vi "Next Background Music.vi"(8 "error in (no error)":errorcluster, 9 "Music Paused":bool, 10 "Dyn Sounds Path":path, 11 "Sounds":T1[](array[typedef]) {"Task ID" format="%.0x"}) -> (0 "error out":errorcluster, 3 "Sounds Out":T1[](array[typedef]) {"Task ID" format="%.0x"}, 5 "BackGround Track":string)   [LabVIEW 2021, in "Sound Manager.lvlib"]
uses:
  Sound Manager.lvlib
  Typedefs/Sound Data.ctl
  Typedefs/Sound Effects.ctl
  <vilib>/sound2/lvsound2.llb/Sound Output Task ID.ctl
  <vilib>/sound2/lvsound2.llb/Sound Output Set Volume (Single).vi
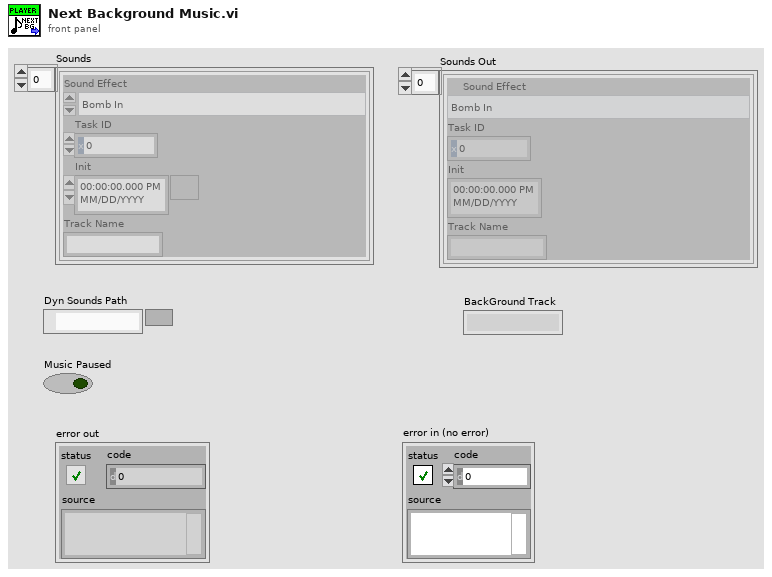
[diagram p1: front panel]
types:
  T1 = typedef "Sound Manager.lvlib/Sound Data.ctl" = cluster{"Sound Effect":T2, "Task ID":T3, "Init":timestamp, "Track Name":string}
  T2 = typedef "Sound Manager.lvlib/Sound Effects.ctl" = enum16{"Bomb In", "Bomb Out", "Bomb Touched", "Game Over", "Victory", "Eat", "10 Fruits", "Eat2", "Eat3", "Eat4", "MaxShield", "Shield", "10p", "Grape In", "Grape Out", "20p", "30p", "40p", "50p", "60p", "70p", "80p", "90p", "100p", "All shields cracked", "Mouse In", "Mouse Out", "Mouse Eaten", "Grape Eaten", "States Recover", "Broken Shield", "Bonus", "Happy Time", "explode", "Game over musica", "Back Music", "Shield Catch", "Evil lough", "Cricket In", "Cricket eaten", "Lets Go", "Jump1", "Jump2", "Jump3", "Unstoppable", "Troll Music", "winner", "menu"}
  T3 = typedef "Sound Output Task ID.ctl" = u32
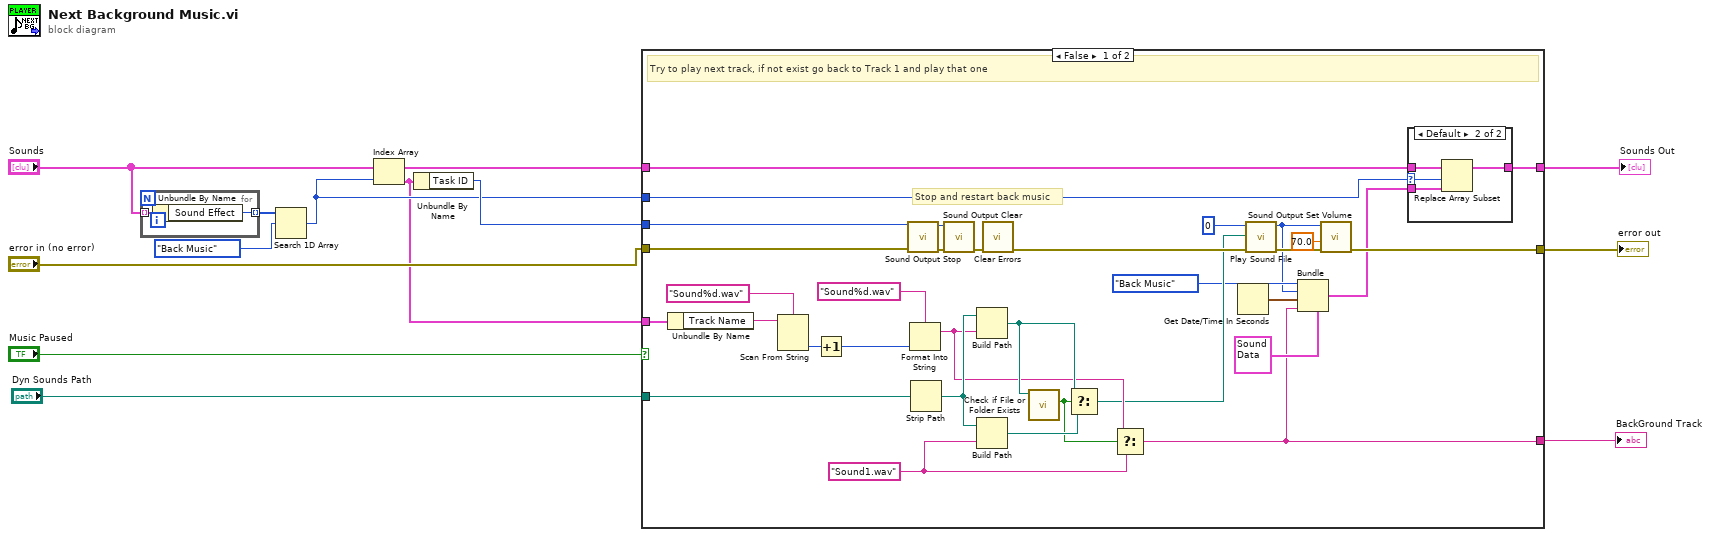
[diagram p0: block diagram]
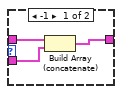
[diagram p2: hidden frame]
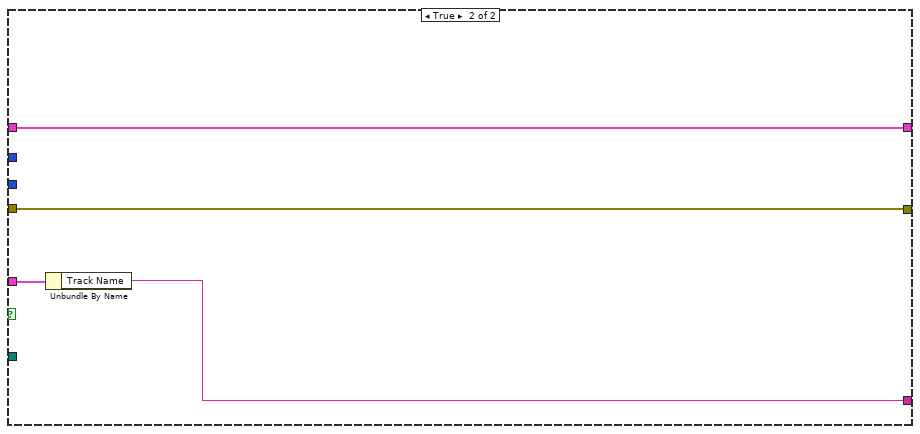
[diagram p3: hidden frame]
diagram:
  n1 = for {
    tunnel: "Sounds" -> [w14] mode=indexing
    tunnel: [w13] -> w11 mode=indexing
    n2 = Unbundle By Name(w14) -> ("Sound Effect"=w13:T2)
  }
  n3 = Search 1D Array(1D array=w11, element=Sound_Effects."Back Music" ("Sound Effect")) -> (index of element=w6:i32)  [unwired: 1 in]
  n4 = Index Array(array="Sounds", index=w6) -> (element=w3:T1)
  n5 = Unbundle By Name(w3) -> ("Task ID"=w12:T3)
  n6 = case shown="False" "Music Paused" {
    tunnel: w12 -> [w45 _]
    tunnel: "error in (no error)" -> [w44 w57]
    tunnel: "Sounds" -> [w42 w58]
    tunnel: [w38 w57] -> w7
    tunnel: w6 -> [w36 _]
    tunnel: [w35 w58] -> w8
    tunnel: "Dyn Sounds Path" -> [w33 _]
    tunnel: [w15 w55] -> w4
    tunnel: w3 -> [w30 w56]
    frame False {
      w21 = "Sound1.wav" ("format string")
      # "Stop and restart back music"
      # "Try to play next track, if not exist go back to Track 1 and play that one"
      n7 = Unbundle By Name(w30) -> ("Track Name"=w28:string)
      n8 = Scan From String(format string="Sound%d.wav", input string=w28) -> (output 1=w27:i32)  [unwired: 3 in, 3 out]
      n9 = Increment(x=w27) -> (x+1=w26:i32)
      n10 = call <vilib>:"Sound Output Stop.vi"("error in (no error)"=w44, "task ID"=w45) -> ("error out"=w43:errorcluster, "task ID out"=w46:T3)  [unwired: 8 in]
      n11 = Format Into String(format string="Sound%d.wav", w26) -> (resulting string=w22:string)  [unwired: 2 in, 1 out]
      n12 = Strip Path(path=w33) -> (stripped path=w24:path)  [unwired: 1 out]
      n13 = call <vilib>:"Sound Output Clear.vi"("error in (no error)"=w43, "task ID"=w46) -> ("error out"=w47:errorcluster)  [unwired: 9 in]
      n14 = Build Path(base path=w24, name or relative path=w22) -> (appended path=w25:path)
      n15 = Build Path(base path=w24, name or relative path=w21) -> (appended path=w23:path)
      n16 = call <vilib>:"Clear Errors.vi"("error in (no error)"=w47) -> ("error out"=w39:errorcluster)  [unwired: 5 in, 1 out]
      n17 = call <vilib>:"Check if File or Folder Exists.vi"("path"=w25) -> ("file or folder exists?"=w20:bool)  [unwired: 8 in, 2 out]
      n18 = Select(t=w25, s=w20, f=w23) -> (s? t:f=w19:path)
      n19 = Select(t=w22, s=w20, f=w21) -> (s? t:f=w15:string)
      n20 = Get Date/Time In Seconds() -> (seconds since 1Jan1904=w18:timestamp)
      n21 = call <vilib>:"Play Sound File.vi"("error in (no error)"=w39, "path"=w19, "device ID"=u32 0) -> ("error out"=w40:errorcluster, "task ID"=w16:T3)  [unwired: 7 in]
      n22 = Bundle(cluster=T1 {"Sound Effect"=enum."Bomb In", "Task ID"=0, "Init"=timestamp(0 s since 1904-01-01), "Track Name"=""} ("Cluster"), "Sound Effect"=Sound_Effects."Back Music", "Task ID"=w16, "Init"=w18, "Track Name"=w15) -> (w37:T1)
      n23 = call-poly <vilib>:"Sound Output Set Volume.vi"("error in (no error)"=w40, "volume"=70.0, "task ID"=w16) -> ("error out"=w38:errorcluster)  [unwired: 7 in, 1 out]
      n24 = case shown="Default" w36 {
        selector: w36 -> [_ w52]
        tunnel: w42 -> [w50 w54]
        tunnel: w37 -> [w48 w53]
        tunnel: [w49 w51] -> w35
        frame -1 {
          n25 = Build Array (concatenate)(w50, w48) -> (w49:T1[])
        }
        frame Default {
          n26 = Replace Array Subset(array=w54, new element=w53, index=w52) -> (w51:T1[])
        }
      }
    }
    frame True {
      n27 = Unbundle By Name(w56) -> ("Track Name"=w55:string)
    }
  }
  "Sounds Out" <- w8
  "error out" <- w7
  "BackGround Track" <- w4
